vi "Obtain top dispatch vi.vi"(8 "Error In":errorcluster, 11 "VI name":string) -> (0 "Error Out":errorcluster, 2 "Found":bool, 3 "vi reference":refnum<vi>)   [LabVIEW 2019]
panel:
  out "element":string
  out "Numeric Control":i32
  out "call chain":string[](array[string])
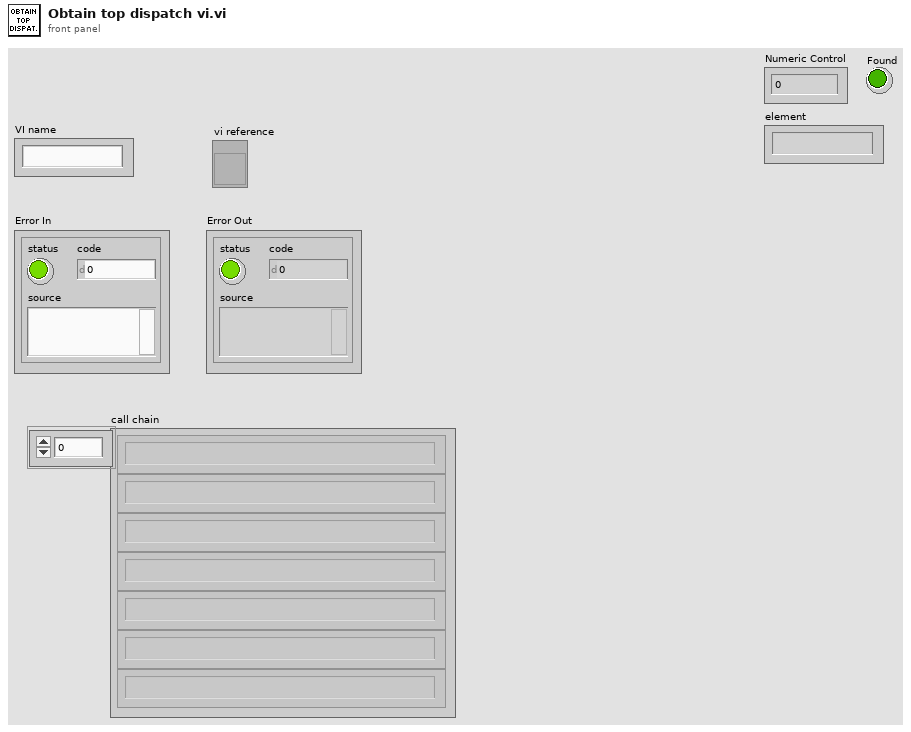
[diagram p1: front panel]
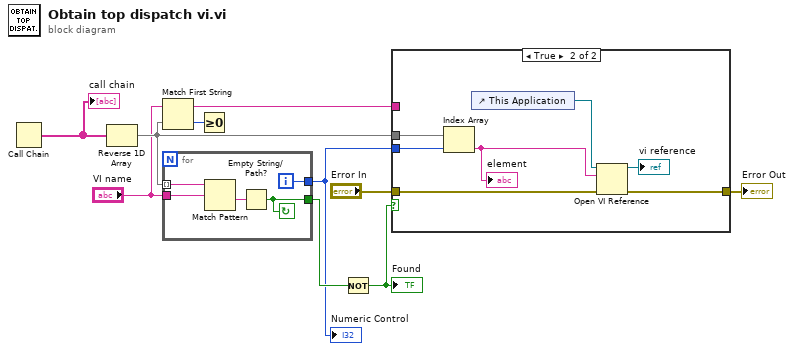
[diagram p0: block diagram]
diagram:
  n1 = Call Chain() -> (call chain=w6:string[])
  "call chain" <- w6
  n2 = Reverse 1D Array(array=w6) -> (reversed array=w5:string[])
  n3 = Match First String(2:w5, 3:"VI name") -> (0:w9:i32, 1:w10:string)
  n4 = for {
    tunnel: w5 -> [w15] mode=indexing
    tunnel: "VI name" -> [w14]
    tunnel: [w12] -> w3
    tunnel: [w11] -> w2
    i -> [w11]
    stop <- w12 continue-if-true
    n5 = Match Pattern(string=w15, regular expression=w14) -> (after substring=w13:string)  [unwired: 1 in, 3 out]
    n6 = Empty String/Path?(string/path=w13) -> (empty?=w12:bool)
  }
  "Numeric Control" <- w2
  n7 = Greater Or Equal To 0?(x=w9) -> ()  [unwired: 1 out]
  n8 = Not(x=w3) -> (.not. x?=w1:bool)
  "Found" <- w1
  n9 = case shown="True" w1 {
    tunnel: w10 -> [_ _]
    tunnel: w5 -> [_ w20]
    tunnel: w2 -> [_ w19]
    tunnel: [w16 w18] -> w8
    tunnel: "Error In" -> [w16 w17]
    frame False {
    }
    frame True {
      n10 = Index Array(array=w20, index=w19) -> (element=w22:string)
      "element" <- w22
      n11 = control-ref of="This Application"() -> (w23:refnum<vi>)
      n12 = Open VI Reference(application reference (local)=w23, vi path=w22, error in (no error)=w17) -> (vi reference=→"vi reference":refnum<vi>, error out=w18:errorcluster)  [unwired: 3 in]
    }
  }
  "Error Out" <- w8
